vi "convertOldSetlist.vi"(0 "HW settings path":path=path "D:/My Documents/NIST (postdoc)/Labview/Data Acquisition/Hardware Control/Hardware/20121128_rbI_default_locked", 1 "Load pre 5.6 Globals?":bool, 5 "Procedure path":path=path "D:/My Documents/NIST (postdoc)/Labview/Data Acquisition/Hardware Control/procedures/201300927_Bzscan_Talbot", 7 "Version Selection":T4(radio)=enum."Load DDS 4.10", 11 "error in":errorcluster) -> (3 "Procedure Name":string, 4 "Devices":refnum<class "Device.lvclass">[](array[class]), 6 "Static Variables":T2[](array[typedef]), 8 "Sequencing Info":T3(array[cluster]), 10 "User defined functions":string, 15 "error out":errorcluster)   [LabVIEW 2013]
uses:
  TypeDefs/Active procedure variables.ctl
  DeviceVIs/DDS/DDS.lvclass
  DeviceVIs/NI Card/NI Card.lvclass
  DeviceVIs/Novatech/Novatech.lvclass
  DeviceVIs/Pulseblaster/Pulseblaster.lvclass
  DeviceVIs/Device/Device.lvclass
  <vilib>/Utility/miscctls.llb/LVStringsAndValuesArrayTypeDef_I32.ctl
panel:
  out "NI Card Trig Lines":u16[](array[numeric])
  out "Novatech Trig Lines":u16[](array[numeric])
  out "DDS Trig Lines":u16[](array[numeric])
  in  "Tab Control":T1(tab)
  in  "Select Layout":i32(ring) items=["Default"]
  out "Final PB Master Table":string[][](array[string])
  out "Final NI Device Table":string[][](array[string])
  out "Final Novatech Channel Table":string[][](array[string])
  out "Final DDS Table":string[][](array[string])
  out "DDS Object Array":refnum<class "DDS.lvclass">[](array[class])
  out "NI Card Array":refnum<class "NI Card.lvclass">[](array[class])
  in  "Master PulseBlaster":refnum<class "Pulseblaster.lvclass">
  out "Novatech Object Array":refnum<class "Novatech.lvclass">[](array[class])
  out "Slave PB Array":refnum<class "Pulseblaster.lvclass">[](array[class])
  out "DDS Devices":T5(array[cluster])
  out "Slave Tables":T6
  out "Master Tables":T6
  out "Novatech Devices":T7(array[cluster])
  out "Novatech Ramps":T8(array[cluster])
  out "NI Cards":T9(array[cluster])
  out "SRS Ramps":T10(array[cluster])
  out "# of DO channels":i32
  out "# of AO channels":i32
  out "# DDS Devices":i32
  out "# Novatech devices":i32
  out "# NI Cards":i32
  out "Length of setlist (lines)":i32
  out "ColHdrs":string[](array[string])
  out "# of AI channels":i32
  # "Debugging:\n\nRight number of rows - YES\nMaster PB - Table = YES\nMaster PB - Hardware?\nDO - Table = Yes \nAO - Table = Yes\nNovatech - ???\nDDS - Table = Yes"
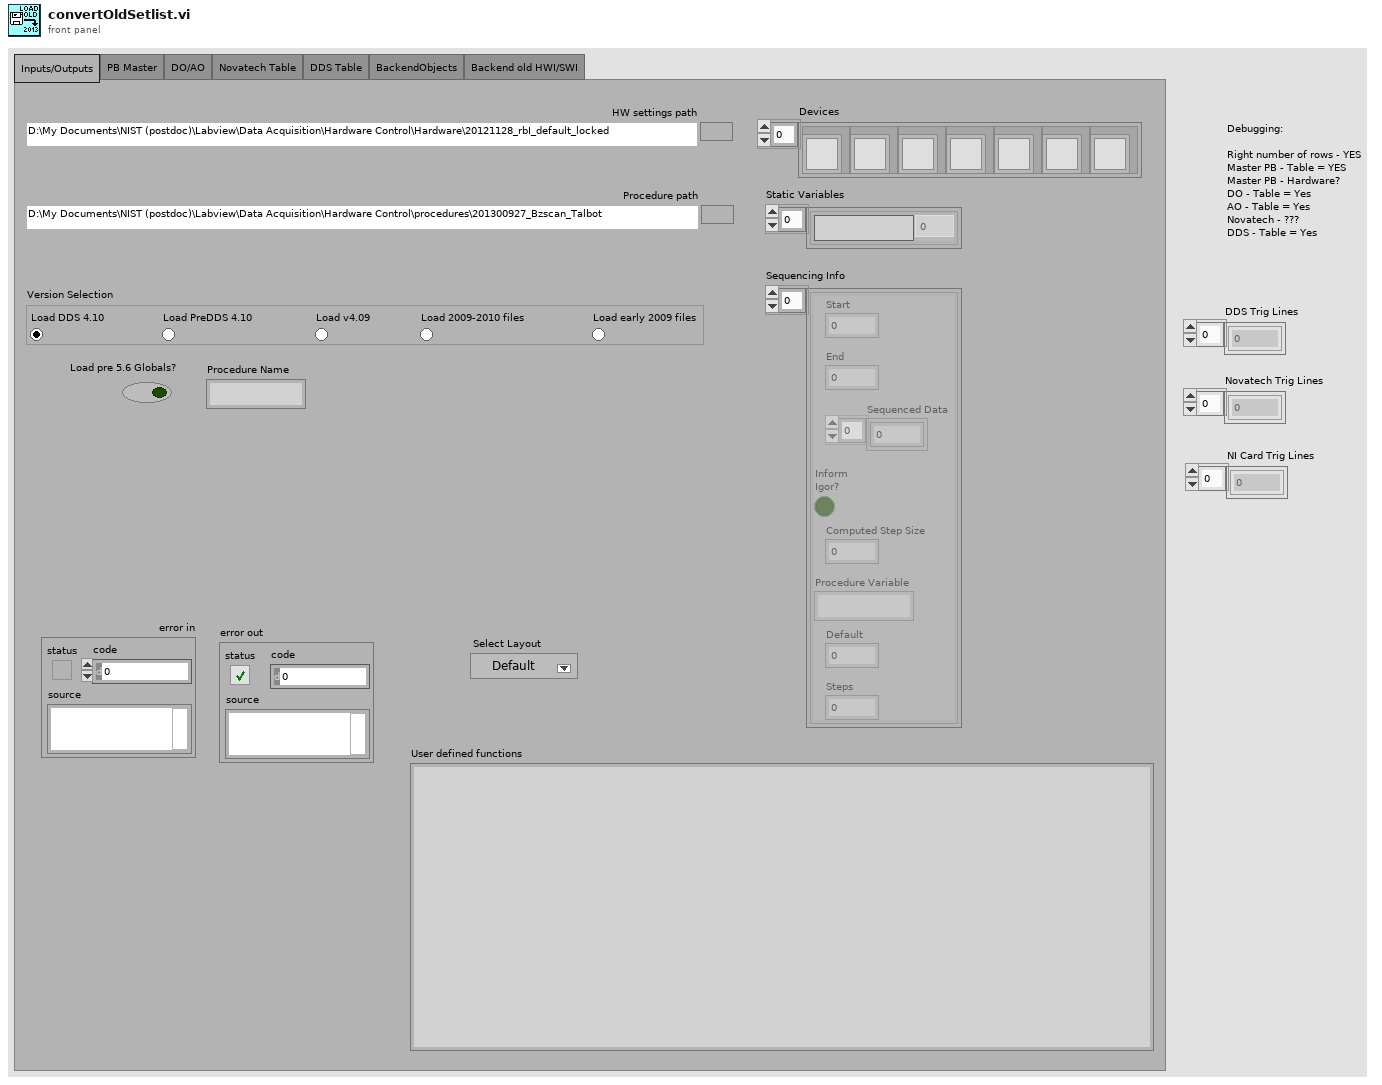
[diagram p1: front panel]
types:
  T1 = enum32{"Inputs/Outputs", "PB Master", "DO/AO", "Novatech Table", "DDS Table", "BackendObjects", "Backend old HWI/SWI"}
  T2 = typedef "Active procedure variables.ctl" = cluster{"Procedure variable":string, "Value":dbl}
  T3 = cluster{"Start":dbl, "End":dbl, "Sequenced Data":dbl[], "Inform\nIgor?":bool, "Computed Step Size":dbl, "Procedure Variable":string, "Default":dbl, "Steps":i32}[]
  T4 = enum32{"Load PreDDS 4.10", "Load early 2009 files", "Load 2009-2010 files", "Load DDS 4.10", "Load v4.09"}
  T5 = cluster{"PB Trigger Line":u16, "Sweeps":bool, "Channel Name":string, "Device Description":string, "PB trig / Sequence":bool, "Amp Lock":bool, "SetList Display":bool[], "FPGA Firmware Version":dbl}[]
  T6 = cluster{"Master Staging List":cluster{"Marker":string, "Mode":enum16{"Continue", "Ramp", "Loop", "EndLoop", "Halt"}, "Output Bits":bool[], "Delay (s)":string, "Ramp Step":dbl, "String":string, "Line Number":string}[], "Master DO Table":cluster{"Output Bits":bool[]}[], "Master AO Table":string[][], "Novatech Table":string[][], "DDS Table":string[][]}
  T7 = cluster{"PB Trigger Line":u16, "Serial Port":refnum<visa-resource-name>, "Channel Names":string[], "SetList Display":bool[][]}[]
  T8 = cluster{"Ramp Channels":cluster{"Time":string, "0 Freq. [MHz]":string, "0 Power [dBm]":string, "1 Freq. [MHz]":string, "1 Power [dBm]":string}[], "2 Freq. [MHz]":string, "2 Power [dBm]":string, "3 Freq. [MHz]":string, "3 Power [dBm]":string, "Serial Port":refnum<visa-resource-name>}[]
  T9 = cluster{"AO Channels":refnum<k21>[], "Trigger terminal":tag, "DO Channel":refnum<k21>, "AI Channels":refnum<k21>[], "PB Trigger Line":u16, "Trigger Mirror":tag, "DO lines":i32, "AO Channel Names":string[], "AI Channel Names":string[], "AI Pause Line":tag, "AI Sample Rate":dbl, "SetList Display":bool[]}[]
  T10 = cluster{"lattice ramp":cluster{"dt":string, "formula":string}[], "Output":cluster{"Time Values":dbl[], dbl[]}[], "SRS Selection":enum16{"1550 Vertical", "Bragg Agilent", "Bragg PTS", "Acc. Intensity"}}[]
  T11 = cluster{"Master PB Staging List":cluster{"Output Bits":bool[], "Delay (s)":string, "String":string, "Halt?":bool}[], "Slave PB Staging List":cluster{"Output Bits":bool[], "Delay (s)":string, "String":string, "Halt?":bool}[], "Novatech Ramps":cluster{"Ramp Channels":cluster{"Time":string, "0 Freq. [MHz]":string, "0 Power [dBm]":string, "1 Freq. [MHz]":string, "1 Power [dBm]":string}[], "2 Freq. [MHz]":string, "2 Power [dBm]":string, "3 Freq. [MHz]":string, "3 Power [dBm]":string, "Serial Port":refnum<visa-resource-name>}[], "Sequencing Info":cluster{"Start":dbl, "End":dbl, "Sequenced Data":dbl[], "Inform\nIgor?":bool, "Computed Step Size":dbl, "Procedure Variable":string, "Default":dbl, "Steps":i32}[], "SRS Ramps":cluster{"lattice ramp":cluster{"dt":string, "formula":string}[], "Output":cluster{"Time Values":dbl[], dbl[]}[], "SRS Selection":enum16{"1550 Vertical", "Bragg Agilent", "Bragg PTS", "Acc. Intensity"}}[], "Master AO Ramp List":cluster{"Ramp index":u32, "Ramp time [s]":string, "Step size [s]":dbl, "Ramp Array":string[], "Output Bits":bool[]}[], "Slave AO Ramp List":cluster{"Ramp index":u32, "Ramp time [s]":string, "Step size [s]":dbl, "Ramp Array":string[], "Output Bits":bool[]}[], "Master Novatech Ramp List":cluster{"Ramp index":u32, "Ramp time [s]":string, "Step size [s]":dbl, "Data Array":string[]}[], "Static Variables":cluster{"Procedure variable":string, "Value":dbl}[], "DDS Ramp List":cluster{"Ramp index":u32, "Ramp time [s]":string, "Step size [s]":dbl, "Data Array":string[]}[]}
  T12 = cluster{"Master PB Staging List":cluster{"Output Bits":bool[], "Delay (s)":string, "String":string, "Halt?":bool}[], "Slave PB Staging List":cluster{"Output Bits":bool[], "Delay (s)":string, "String":string, "Halt?":bool}[], "Novatech Ramps":cluster{"Ramp Channels":cluster{"Time":string, "0 Freq. [MHz]":string, "0 Power [dBm]":string, "1 Freq. [MHz]":string, "1 Power [dBm]":string}[], "2 Freq. [MHz]":string, "2 Power [dBm]":string, "3 Freq. [MHz]":string, "3 Power [dBm]":string, "Serial Port":refnum<visa-resource-name>}[], "Sequencing Info":cluster{"Start":dbl, "End":dbl, "Sequenced Data":dbl[], "Inform\nIgor?":bool, "Computed Step Size":dbl, "Procedure Variable":string, "Default":dbl, "Steps":i32}[], "SRS Ramps":cluster{"lattice ramp":cluster{"dt":string, "formula":string}[], "Output":cluster{"Time Values":dbl[], dbl[]}[], "SRS Selection":enum16{"1550 Vertical", "Bragg Agilent", "Bragg PTS", "Acc. Intensity"}}[], "Master AO Ramp List":cluster{"Ramp index":u32, "Ramp time [s]":string, "Step size [s]":dbl, "Ramp Array":string[], "Output Bits":bool[]}[], "Slave AO Ramp List":cluster{"Ramp index":u32, "Ramp time [s]":string, "Step size [s]":dbl, "Ramp Array":string[], "Output Bits":bool[]}[], "Master Novatech Ramp List":cluster{"Ramp index":u32, "Ramp time [s]":string, "Step size [s]":dbl, "Data Array":string[]}[], "Static Variables":T2[], "DDS Ramp List":cluster{"Ramp index":u32, "Ramp time [s]":string, "Step size [s]":dbl, "Data Array":string[]}[]}
  T13 = cluster{"User defined functions":string, "Master AO Channels":cluster{"AO Channels":refnum<k21>[], "Trigger terminal":tag, "DO Channel":refnum<k21>, "AI Channels":refnum<k21>[], "PB Trigger Line":u16, "Trigger Mirror":tag, "DO lines":i32, "AO Channel Names":string[], "AI Channel Names":string[], "AI Pause Line":tag, "AI Sample Rate":dbl, "SetList Display":bool[]}[], "Novatech Devices":cluster{"PB Trigger Line":u16, "Serial Port":refnum<visa-resource-name>, "Channel Names":string[], "SetList Display":bool[][]}[], "DDS Devices":cluster{"PB Trigger Line":u16, "Sweeps":bool, "Channel Name":string, "Device Description":string, "PB trig / Sequence":bool, "Amp Lock":bool, "SetList Display":bool[], "FPGA Firmware Version":dbl}[]}
  T14 = typedef "LVStringsAndValuesArrayTypeDef_I32.ctl" = cluster{"String":string, "Value":i32}[]
  T15 = cluster{"Output Bits":bool[], "Delay (s)":string, "String":string, "Halt?":bool}[]
  T16 = cluster{"Ramp index":u32, "Ramp time [s]":string, "Step size [s]":dbl, "Ramp Array":string[], "Output Bits":bool[]}[]
  T17 = cluster{"Ramp index":u32, "Ramp time [s]":string, "Step size [s]":dbl, "Data Array":string[]}[]
  T18 = cluster{"Marker":string, "Mode":enum16{"Continue", "Ramp", "Loop", "EndLoop", "Halt"}, "Output Bits":bool[], "Delay (s)":string, "Ramp Step":dbl, "String":string, "Line Number":string}[]
  T19 = enum16{"Continue", "Ramp", "Loop", "EndLoop", "Halt"}
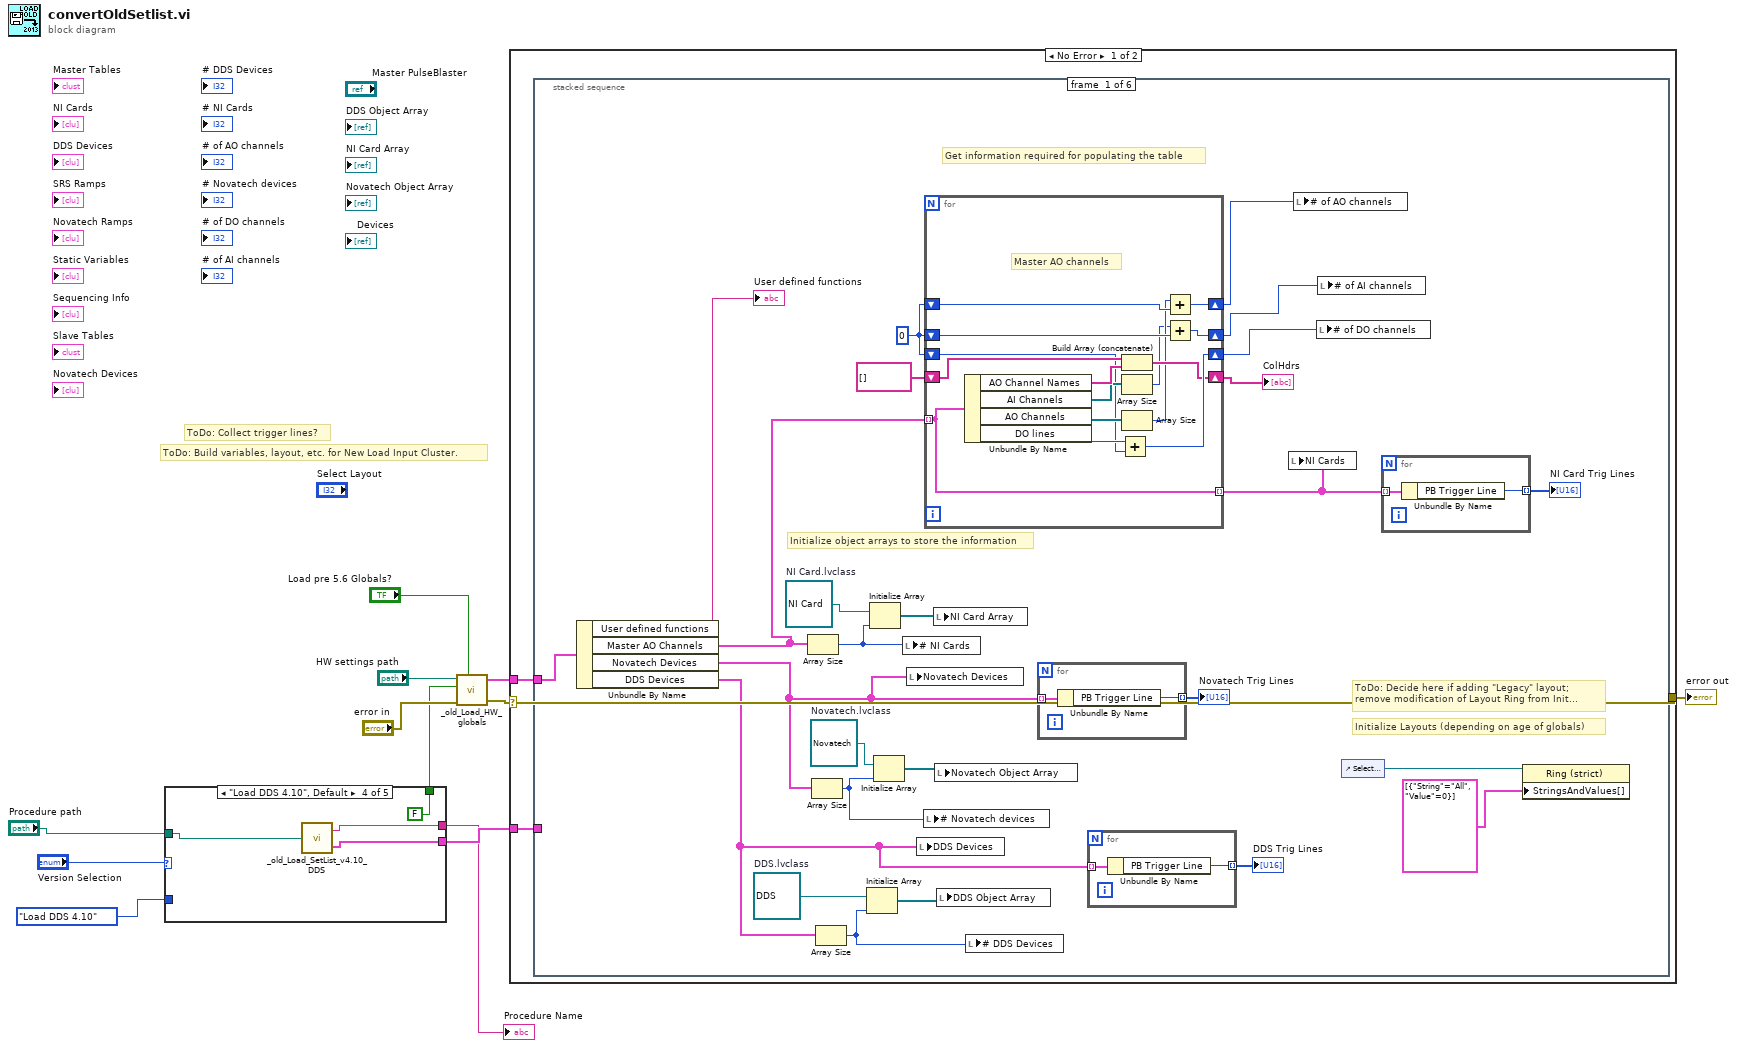
[diagram p0: block diagram]
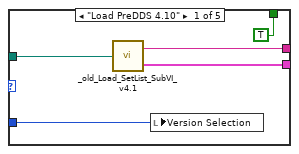
[diagram p2: hidden frame]
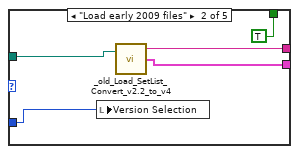
[diagram p3: hidden frame]
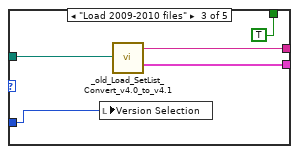
[diagram p4: hidden frame]
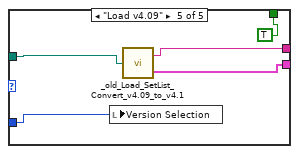
[diagram p5: hidden frame]
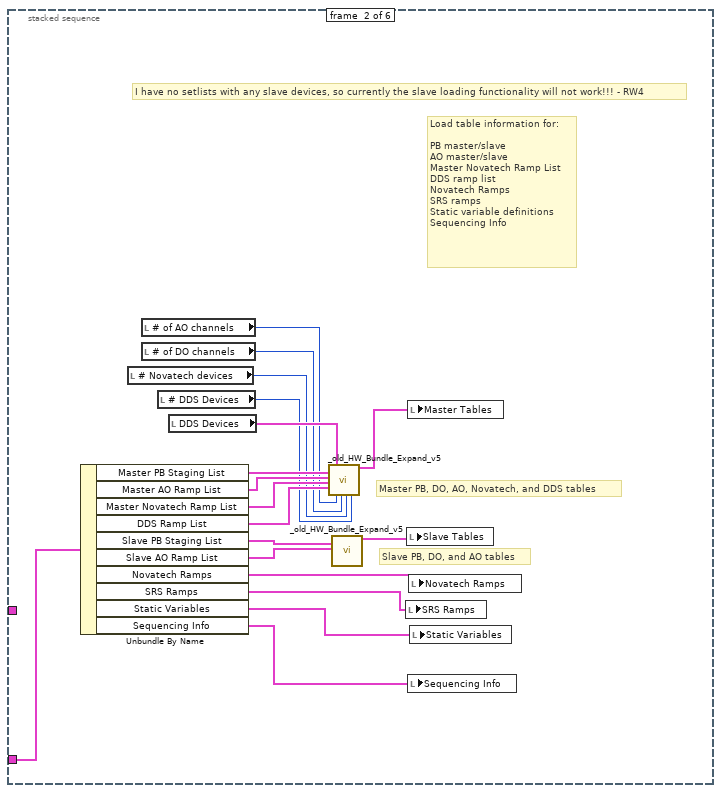
[diagram p6: hidden frame]
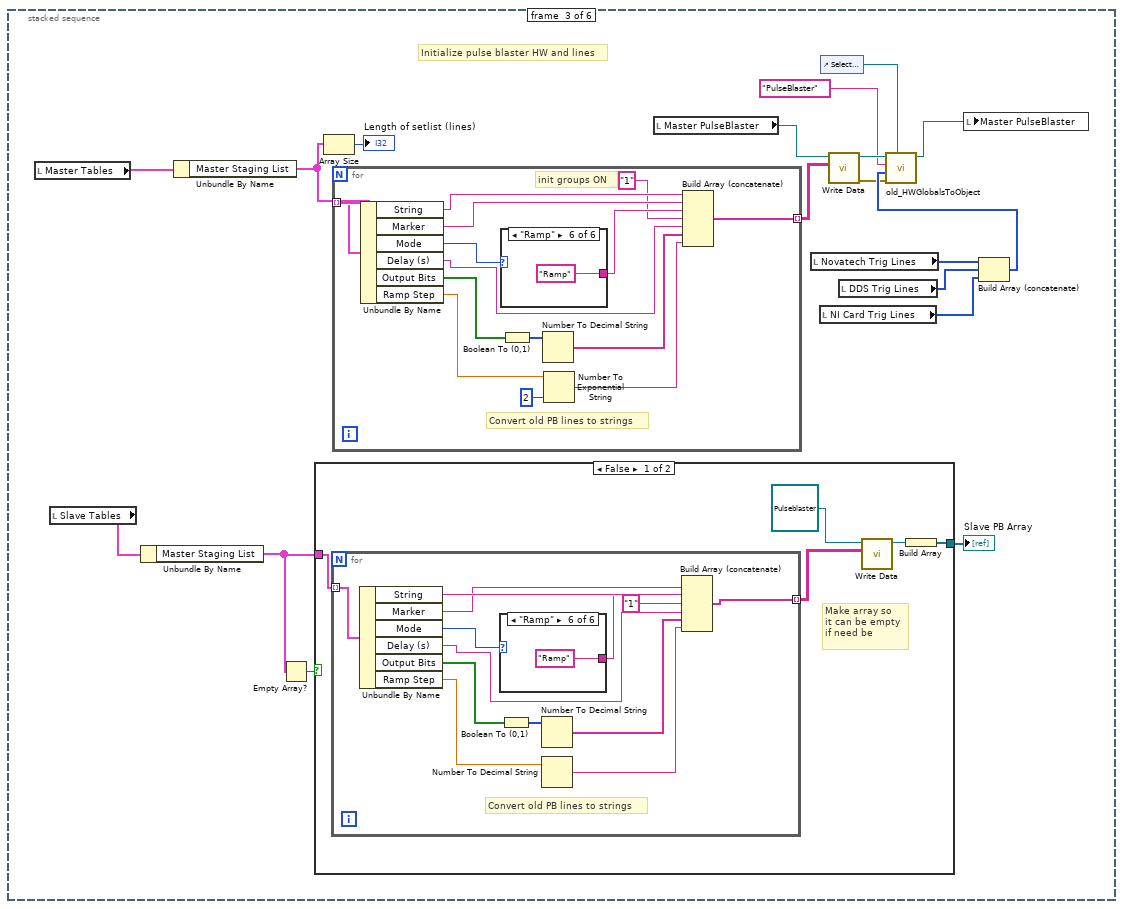
[diagram p7: hidden frame]
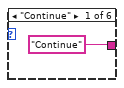
[diagram p8: hidden frame]
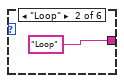
[diagram p9: hidden frame]
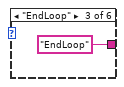
[diagram p10: hidden frame]
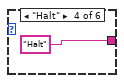
[diagram p11: hidden frame]
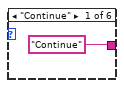
[diagram p14: hidden frame]
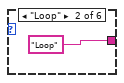
[diagram p15: hidden frame]
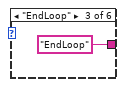
[diagram p16: hidden frame]
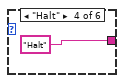
[diagram p17: hidden frame]
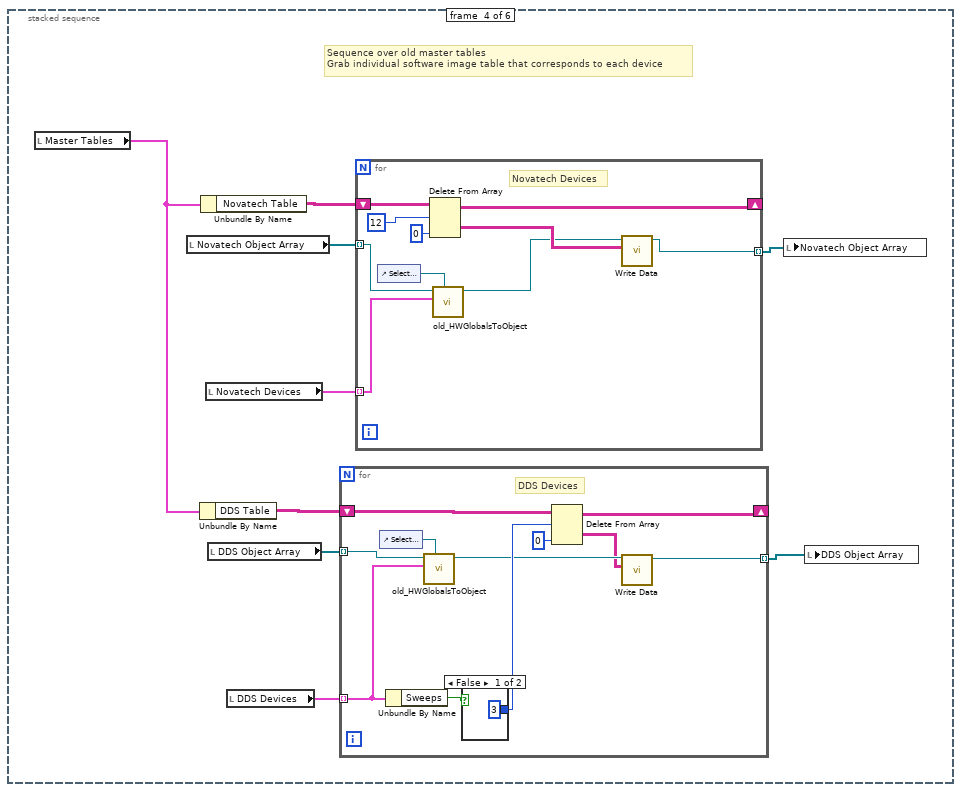
[diagram p19: hidden frame]
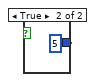
[diagram p20: hidden frame]
diagram:
  # "ToDo: Collect trigger lines?"
  # "ToDo: Build variables, layout, etc. for New Load Input Cluster."
  n1 = case shown="\"Load DDS 4.10\", Default" "Version Selection" {
    tunnel: [w17 w21 w27 w30 w33] -> w4
    tunnel: "Procedure path" -> [w16 w22 w25 w31 w34]
    tunnel: [w15 w20 w26 w29 w32] -> w5
    tunnel: T4."Load DDS 4.10" ("Version Selection") -> [w14 w19 w24 _ w36]
    tunnel: [TRUE TRUE TRUE FALSE TRUE] -> w2
    frame "Load PreDDS 4.10" {
      n2 = call "_old_Load_SetList_SubVI_v4.1.vi"("Path"=w16) -> ("Procedure Name"=w17:string, "Paramaters"=w15:T11)
      n3 = local write "Version Selection"(w14) -> ()
    }
    frame "Load early 2009 files" {
      n4 = local write "Version Selection"(w19) -> ()
      n5 = call "_old_Load_SetList_Convert_v2.2_to_v4.vi"("Path"=w22) -> ("Procedure Name"=w21:string, "Paramaters"=w20:T11)  [unwired: 1 in, 1 out]
    }
    frame "Load 2009-2010 files" {
      n6 = local write "Version Selection"(w24) -> ()
      n7 = call "_old_Load_SetList_Convert_v4.0_to_v4.1.vi"("Path"=w25) -> ("Procedure Name"=w27:string, "Paramaters"=w26:T11)
    }
    frame "Load DDS 4.10", Default {
      n8 = call "_old_Load_SetList_v4.10_DDS.vi"("Path"=w31) -> ("Procedure Name"=w30:string, "Paramaters"=w29:T12)
    }
    frame "Load v4.09" {
      n9 = local write "Version Selection"(w36) -> ()
      n10 = call "_old_Load_SetList_Convert_v4.09_to_v4.1.vi"("Path"=w34) -> ("Procedure Name"=w33:string, "Paramaters"=w32:T11)
    }
  }
  "Procedure Name" <- w4
  n11 = call "_old_Load_HW_globals.vi"("HW settings path"="HW settings path", "Load pre 5.6 Globals?"="Load pre 5.6 Globals?", "Pre 4.1 HWGlobals?"=w2, "error in"="error in") -> ("Loaded Procedure Data"=w12:T13, "error out"=w1:errorcluster)  [unwired: 2 in, 1 out]
  n12 = case shown="No Error" w1 {
    selector: w1 -> [w37 w254]
    tunnel: w5 -> [w38 _]
    tunnel: w12 -> [w39 _]
    tunnel: [w37 w254] -> w8
    frame No Error {
      n13 = stacked-sequence {
        tunnel: w39 -> [w65 _ _ _ _ _]
        tunnel: w38 -> [_ w104 _ _ _ _]
        frame #0 {
          w55 = refnum<class "Novatech.lvclass"> refnum  # Novatech.lvclass
          w56 = refnum<class "NI Card.lvclass"> refnum  # NI Card.lvclass
          w57 = refnum<class "DDS.lvclass"> refnum  # DDS.lvclass
          w62 = 0
          # "ToDo: Decide here if adding \"Legacy\" layout;\nremove modification of Layout Ring from Init..."
          # "Initialize Layouts (depending on age of globals)"
          # "Initialize object arrays to store the information"
          # "Get information required for populating the table"
          n14 = Unbundle By Name(w65) -> ("User defined functions"=→"User defined functions":string, "Master AO Channels"=w61:T9, "Novatech Devices"=w43:T7, "DDS Devices"=w41:T5)
          n15 = Array Size(array=w61) -> (size(s)=w51:i32)
          n16 = Array Size(array=w43) -> (size(s)=w48:i32)
          n17 = Array Size(array=w41) -> (size(s)=w49:i32)
          n18 = Initialize Array(w57, w49) -> (w52:refnum<class "DDS.lvclass">[])
          n19 = Initialize Array(w56, w51) -> (w54:refnum<class "NI Card.lvclass">[])
          n20 = Initialize Array(w55, w48) -> (w53:refnum<class "Novatech.lvclass">[])
          n21 = local write "# NI Cards"(w51) -> ()
          n22 = local write "Novatech Devices"(w43) -> ()
          n23 = local write "DDS Devices"(w41) -> ()
          n24 = local write "# Novatech devices"(w48) -> ()
          n25 = for {
            tunnel: w61 -> [w75] mode=indexing
            shift-right: [w84] -> w59
            shift-left: w62 -> [w73]
            shift-right: [w83] -> w58
            shift-left: w62 -> [w85]
            shift-right: [w82] -> w60
            shift-left: w62 -> [w86]
            shift-right: [w78] -> w63
            shift-left: string[] [] ("initialized array") -> [w79]
            tunnel: [w75] -> w45 mode=indexing
            # "Master AO channels"
            n26 = Unbundle By Name(w75) -> ("AO Channel Names"=w80:string[], "AI Channels"=w77:refnum<k21>[], "AO Channels"=w76:refnum<k21>[], "DO lines"=w81:i32)
            n27 = Add(x=w81, y=w73) -> (x+y=w84:i32)
            n28 = Build Array (concatenate)(w79, w80) -> (w78:string[])
            n29 = Array Size(array=w77) -> (size(s)=w72:i32)
            n30 = Array Size(array=w76) -> (size(s)=w74:i32)
            n31 = Add(x=w74, y=w86) -> (x+y=w82:i32)
            n32 = Add(x=w72, y=w85) -> (x+y=w83:i32)
          }
          "ColHdrs" <- w63
          n33 = local write "NI Card Array"(w54) -> ()
          n34 = local write "Novatech Object Array"(w53) -> ()
          n35 = local write "DDS Object Array"(w52) -> ()
          n36 = local write "# DDS Devices"(w49) -> ()
          n37 = for {
            tunnel: w43 -> [w69] mode=indexing
            tunnel: [w68] -> w42 mode=indexing
            n38 = Unbundle By Name(w69) -> ("PB Trigger Line"=w68:u16)
          }
          "Novatech Trig Lines" <- w42
          n39 = for {
            tunnel: w41 -> [w67] mode=indexing
            tunnel: [w66] -> w40 mode=indexing
            n40 = Unbundle By Name(w67) -> ("PB Trigger Line"=w66:u16)
          }
          "DDS Trig Lines" <- w40
          n41 = local write "NI Cards"(w45) -> ()
          n42 = local write "# of AO channels"(w60) -> ()
          n43 = local write "# of DO channels"(w59) -> ()
          n44 = local write "# of AI channels"(w58) -> ()
          n45 = control-ref of="Select Layout"() -> (w47:refnum<vi>)
          n46 = for {
            tunnel: w45 -> [w71] mode=indexing
            tunnel: [w70] -> w44 mode=indexing
            n47 = Unbundle By Name(w71) -> ("PB Trigger Line"=w70:u16)
          }
          "NI Card Trig Lines" <- w44
          n48 = property class="Ring (strict)"(reference=w47, "StringsAndValues[]"=T14 [{"String"="All", "Value"=0}] ("Strings And Values []")) -> ()  [unwired: 1 in, 2 out]
        }
        frame #1 {
          # "I have no setlists with any slave devices, so currently the slave loading functionality will not work!!! - RW4"
          # "Load table information for:\n\nPB master/slave\nAO master/slave\nMaster Novatech Ramp List\nDDS ramp list\nNovatech Ramps\nSRS ramps\nStatic variable definitions\nSequencing Info"
          # "Slave PB, DO, and AO tables"
          # "Master PB, DO, AO, Novatech, and DDS tables"
          n49 = Unbundle By Name(w104) -> ("Master PB Staging List"=w103:T15, "Master AO Ramp List"=w102:T16, "Master Novatech Ramp List"=w101:T17, "DDS Ramp List"=w100:T17, "Slave PB Staging List"=w98:T15, "Slave AO Ramp List"=w97:T16, "Novatech Ramps"=w95:T8, "SRS Ramps"=w96:T10, "Static Variables"=w93:T2[], "Sequencing Info"=w94:T3)
          n50 = local read "# Novatech devices"() -> (w88:i32)
          n51 = local read "# of AO channels"() -> (w90:i32)
          n52 = local read "# of DO channels"() -> (w89:i32)
          n53 = local read "# DDS Devices"() -> (w87:i32)
          n54 = local read "DDS Devices"() -> (w99:T5)
          n55 = call "_old_HW_Bundle_Expand_v5.vi"("PB Staging List"=w103, "AO Ramp List"=w102, "Novatech Ramp List"=w101, "DDS Ramp List"=w100, "DDS Devices"=w99, "Number of AO channels"=w90, "Number of DO channels"=w89, "Number of Novatech channels"=w88, "Number of DDS channels"=w87) -> ("Master Tables"=w92:T6)  [unwired: 10 in]
          n56 = call "_old_HW_Bundle_Expand_v5.vi"("PB Staging List"=w98, "AO Ramp List"=w97) -> ("Master Tables"=w91:T6)  [unwired: 17 in]
          n57 = local write "SRS Ramps"(w96) -> ()
          n58 = local write "Slave Tables"(w91) -> ()
          n59 = local write "Master Tables"(w92) -> ()
          n60 = local write "Sequencing Info"(w94) -> ()
          n61 = local write "Novatech Ramps"(w95) -> ()
          n62 = local write "Static Variables"(w93) -> ()
        }
        frame #2 {
          # "Initialize pulse blaster HW and lines"
          n63 = local read "Master Tables"() -> (w122:T6)
          n64 = local read "Slave Tables"() -> (w117:T6)
          n65 = Unbundle By Name(w117) -> ("Master Staging List"=w116:T18)
          n66 = Unbundle By Name(w122) -> ("Master Staging List"=w120:T18)
          n67 = Empty Array?(array=w116) -> (empty?=w115:bool)
          n68 = case shown="False" w115 {
            tunnel: w116 -> [w126 _]
            tunnel: [w124 _] -> w114
            frame False {
              # "Make array so\nit can be empty\nif need be"
              n69 = for {
                tunnel: w126 -> [w140] mode=indexing
                tunnel: [w132] -> w127 mode=indexing
                # "Convert old PB lines to strings"
                n70 = Unbundle By Name(w140) -> ("String"=w139:string, "Marker"=w138:string, "Mode"=w137:T19, "Delay (s)"=w129:string, "Output Bits"=w134:bool[], "Ramp Step"=w135:dbl)
                n71 = case shown="\"Ramp\"" w137 {
                  tunnel: ["Continue" "Loop" "EndLoop" "Halt" _ "Ramp"] -> w136
                  frame "Continue" {
                  }
                  frame "Loop" {
                  }
                  frame "EndLoop" {
                  }
                  frame "Halt" {
                  }
                  frame Default {
                  }
                  frame "Ramp" {
                  }
                }
                n72 = Boolean To (0,1)(Boolean=w134) -> (0, 1=w133:i16[])
                n73 = Number To Decimal String(number=w133) -> (decimal integer string=w130:string[])  [unwired: 1 in]
                n74 = Number To Decimal String(number=w135) -> (decimal integer string=w131:string)  [unwired: 1 in]
                n75 = Build Array (concatenate)(w139, w138, w136, "1" ("element"), w129, w130, w131) -> (w132:string[])
              }
              n76 = call-dynamic "Write Data.vi"("Data"=w127, "Device in"=refnum<class "Pulseblaster.lvclass"> refnum ("Master PulseBlaster")) -> ("Device Out"=w125:refnum<class "Pulseblaster.lvclass">)  [unwired: 8 in, 1 out]
              n77 = Build Array(w125) -> (w124:refnum<class "Pulseblaster.lvclass">[])
            }
            frame True {
              # "No Slave PB"
            }
          }
          "Slave PB Array" <- w114
          n78 = Array Size(array=w120) -> (size(s)=→"Length of setlist (lines)":i32)
          n79 = for {
            tunnel: w120 -> [w159] mode=indexing
            tunnel: [w152] -> w119 mode=indexing
            # "init groups ON"
            # "Convert old PB lines to strings"
            n80 = Unbundle By Name(w159) -> ("String"=w158:string, "Marker"=w157:string, "Mode"=w156:T19, "Delay (s)"=w150:string, "Output Bits"=w154:bool[], "Ramp Step"=w147:dbl)
            n81 = case shown="\"Ramp\"" w156 {
              tunnel: ["Continue" "Loop" "EndLoop" "Halt" _ "Ramp"] -> w155
              frame "Continue" {
              }
              frame "Loop" {
              }
              frame "EndLoop" {
              }
              frame "Halt" {
              }
              frame Default {
              }
              frame "Ramp" {
              }
            }
            n82 = Boolean To (0,1)(Boolean=w154) -> (0, 1=w153:i16[])
            n83 = Number To Decimal String(number=w153) -> (decimal integer string=w151:string[])  [unwired: 1 in]
            n84 = Number To Exponential String(number=w147, precision (6)=i16 2) -> (E-format string=w148:string)  [unwired: 2 in]
            n85 = Build Array (concatenate)(w158, w157, w155, "1" ("element"), w150, w151, w148) -> (w152:string[])
          }
          n86 = local read "Master PulseBlaster"() -> (w118:refnum<class "Pulseblaster.lvclass">)
          n87 = local read "Novatech Trig Lines"() -> (w110:u16[])
          n88 = local read "NI Card Trig Lines"() -> (w108:u16[])
          n89 = control-ref of="Select Layout"() -> (w105:refnum<vi>)
          n90 = call-dynamic "Write Data.vi"("Data"=w119, "Device in"=w118) -> ("error out"=w106:errorcluster, "Device Out"=w113:refnum<class "Pulseblaster.lvclass">)  [unwired: 8 in]
          n91 = local read "DDS Trig Lines"() -> (w109:u16[])
          n92 = Build Array (concatenate)(w110, w109, w108) -> (w107:u16[])
          n93 = call "old_HWGlobalsToObject.vi"("Select Layout"=w105, "error in (no error)"=w106, "Trigger Lines"=w107, "Name"="PulseBlaster", "Pulseblaster in"=w113) -> ("Pulseblaster out"=w112:refnum<class "Pulseblaster.lvclass">)  [unwired: 5 in, 1 out]
          n94 = local write "Master PulseBlaster"(w112) -> ()
        }
        frame #3 {
          # "Sequence over old master tables\nGrab individual software image table that corresponds to each device"
          n95 = local read "Master Tables"() -> (w165:T6)
          n96 = local read "Novatech Object Array"() -> (w166:refnum<class "Novatech.lvclass">[])
          n97 = Unbundle By Name(w165) -> ("DDS Table"=w171:string[][])
          n98 = Unbundle By Name(w165) -> ("Novatech Table"=w168:string[][])
          n99 = local read "Novatech Devices"() -> (w167:T7)
          n100 = local read "DDS Object Array"() -> (w173:refnum<class "DDS.lvclass">[])
          n101 = local read "DDS Devices"() -> (w172:T5)
          n102 = for {
            tunnel: w173 -> [w188] mode=indexing
            tunnel: w172 -> [w186] mode=indexing
            shift-right: [w189] -> _
            shift-left: w171 -> [w193]
            tunnel: [w190] -> w170 mode=indexing
            # "DDS Devices"
            n103 = control-ref of="Select Layout"() -> (w184:refnum<vi>)
            n104 = Unbundle By Name(w186) -> ("Sweeps"=w194:bool)
            n105 = call "old_HWGlobalsToObject.vi"("Select Layout"=w184, "DDS Device"=w186, "DDS in"=w188) -> ("DDS out"=w187:refnum<class "DDS.lvclass">)  [unwired: 7 in, 1 out]
            n106 = case shown="False" w194 {
              tunnel: [3 5] -> w191
              frame False {
              }
              frame True {
              }
            }
            n107 = Delete From Array(array=w193, length=w191, index (col)=0 ("disabled index (col)")) -> (deleted portion=w185:string[][], array with subset deleted=w189:string[][])  [unwired: 1 in]
            n108 = call-dynamic "Write Data.vi"("Data"=w185, "Device in"=w187) -> ("Device Out"=w190:refnum<class "DDS.lvclass">)  [unwired: 8 in, 1 out]
          }
          n109 = for {
            tunnel: w166 -> [w177] mode=indexing
            tunnel: w167 -> [w175] mode=indexing
            shift-right: [w182] -> _
            shift-left: w168 -> [w183]
            tunnel: [w179] -> w169 mode=indexing
            # "Novatech Devices"
            n110 = control-ref of="Select Layout"() -> (w174:refnum<vi>)
            n111 = Delete From Array(array=w183, length=12, index (col)=0 ("disabled index (col)")) -> (deleted portion=w178:string[][], array with subset deleted=w182:string[][])  [unwired: 1 in]
            n112 = call "old_HWGlobalsToObject.vi"("Select Layout"=w174, "Novatech Channel"=w175, "Novatech in"=w177) -> ("Novatech out"=w176:refnum<class "Novatech.lvclass">)  [unwired: 7 in, 1 out]
            n113 = call-dynamic "Write Data.vi"("Data"=w178, "Device in"=w176) -> ("Device Out"=w179:refnum<class "Novatech.lvclass">)  [unwired: 8 in, 1 out]
          }
          n114 = local write "Novatech Object Array"(w169) -> ()
          n115 = local write "DDS Object Array"(w170) -> ()
        }
        frame #4 {
          # "Sequence over NI card devices... take extra care because of AO/DO lines. DO come first in the final string table"
          # "Method to write\nhardware data"
          # "Method\nto write\ndata"
          n116 = local read "Master Tables"() -> (w202:T6)
          n117 = Unbundle By Name(w202) -> ("Master AO Table"=w201:string[][], "Master DO Table"=w200:cluster{"Output Bits":bool[]}[])
          n118 = for {
            tunnel: [w205] -> w199 mode=indexing
            tunnel: w200 -> [w204] mode=indexing
            n119 = Unbundle By Name(w204) -> ("Output Bits"=w207:bool[])
            n120 = Boolean To (0,1)(Boolean=w207) -> (0, 1=w206:i16[])
            n121 = Number To Decimal String(number=w206) -> (decimal integer string=w205:string[])  [unwired: 1 in]
          }
          n122 = local read "NI Card Array"() -> (w197:refnum<class "NI Card.lvclass">[])
          n123 = local read "NI Cards"() -> (w203:T9)
          n124 = for {
            shift-right: [w220] -> _
            shift-left: w201 -> [w226]
            tunnel: w203 -> [w216] mode=indexing
            shift-right: [w221] -> _
            shift-left: w199 -> [w223]
            tunnel: [w217] -> w198 mode=indexing
            tunnel: w197 -> [w215] mode=indexing
            # "init apperance cols"
            # "DOs first!"
            # "NI Card Devices"
            n125 = Unbundle By Name(w216) -> ("AO Channels"=w222:refnum<k21>[], "DO lines"=w211:i32)
            n126 = control-ref of="Select Layout"() -> (w208:refnum<vi>)
            n127 = call "old_HWGlobalsToObject.vi"("Select Layout"=w208, "Master AO Channel"=w216, "NI Card in"=w215) -> ("error out"=w209:errorcluster, "NI Card out"=w210:refnum<class "NI Card.lvclass">)  [unwired: 7 in]
            n128 = Array Size(array=w222) -> (size(s)=w212:i32)
            n129 = Delete From Array(array=w223, length=w211, index (col)=0 ("disabled index (col)")) -> (deleted portion=w213:string[][], array with subset deleted=w221:string[][])  [unwired: 1 in]
            n130 = Delete From Array(array=w226, length=w212, index (col)=0 ("disabled index (col)")) -> (deleted portion=w214:string[][], array with subset deleted=w220:string[][])  [unwired: 1 in]
            n131 = Insert Into Array(array=w214, index (col)=0 ("disabled index (col)"), new element=w213) -> (w218:string[][])  [unwired: 1 in]
            n132 = call-dynamic "Write Data.vi"("error in (no error)"=w209, "Data"=w218, "Device in"=w210) -> ("Device Out"=w217:refnum<class "NI Card.lvclass">)  [unwired: 7 in, 1 out]
          }
          n133 = local write "NI Card Array"(w198) -> ()
        }
        frame #5 {
          # "Store final device object array"
          n134 = local read "Master PulseBlaster"() -> (w241:refnum<class "Pulseblaster.lvclass">)
          n135 = local read "Novatech Object Array"() -> (w237:refnum<class "Novatech.lvclass">[])
          n136 = local read "DDS Object Array"() -> (w236:refnum<class "DDS.lvclass">[])
          n137 = local read "NI Card Array"() -> (w238:refnum<class "NI Card.lvclass">[])
          n138 = Build Array(w241) -> (w239:refnum<class "Pulseblaster.lvclass">[])
          n139 = Insert Into Array(array=refnum<class "Device.lvclass">[] [] ("Devices 2"), new element #1=w239, new element #2=w238, new element #3=w237, new element #4=w236) -> (w240:refnum<class "Device.lvclass">[])  [unwired: 1 in]
          n140 = local write "Devices"(w240) -> ()
          n141 = for {
            tunnel: w239 -> [w253] mode=indexing
            tunnel: [w251] -> w235 mode=concatenating
            # "PB Master"
            n142 = call-dynamic "Get Data.vi"("Device in"=w253) -> ("Table Indicator"=w252:string[][])  [unwired: 7 in, 2 out]
            n143 = Transpose 2D Array(2D array=w252) -> (transposed array=w251:string[][])
          }
          n144 = for {
            tunnel: [w245] -> w230 mode=concatenating
            tunnel: w237 -> [w247] mode=indexing
            # "Novatech"
            n145 = call-dynamic "Get Data.vi"("Device in"=w247) -> ("Table Indicator"=w246:string[][])  [unwired: 7 in, 2 out]
            n146 = Transpose 2D Array(2D array=w246) -> (transposed array=w245:string[][])
          }
          n147 = for {
            tunnel: [w248] -> w232 mode=concatenating
            tunnel: w238 -> [w250] mode=indexing
            # "NI Card"
            n148 = call-dynamic "Get Data.vi"("Device in"=w250) -> ("Table Indicator"=w249:string[][])  [unwired: 7 in, 2 out]
            n149 = Transpose 2D Array(2D array=w249) -> (transposed array=w248:string[][])
          }
          n150 = for {
            tunnel: [w242] -> w228 mode=concatenating
            tunnel: w236 -> [w244] mode=indexing
            # "DDS"
            n151 = call-dynamic "Get Data.vi"("Device in"=w244) -> ("Table Indicator"=w243:string[][])  [unwired: 7 in, 2 out]
            n152 = Transpose 2D Array(2D array=w243) -> (transposed array=w242:string[][])
          }
          n153 = Transpose 2D Array(2D array=w235) -> (transposed array=→"Final PB Master Table":string[][])
          n154 = Transpose 2D Array(2D array=w228) -> (transposed array=→"Final DDS Table":string[][])
          n155 = Transpose 2D Array(2D array=w230) -> (transposed array=→"Final Novatech Channel Table":string[][])
          n156 = Transpose 2D Array(2D array=w232) -> (transposed array=→"Final NI Device Table":string[][])
        }
      }
    }
    frame Error {
    }
  }
  "error out" <- w8
